vi "while循环的移位寄存器使用.vi"() -> ()   [LabVIEW 2019]
panel:
  out "数组 2":i32[](array[numeric])
  out "数组":i32[](array[numeric])
  out "数值 3":i32
  out "数值 2":i32
  out "数值":i32
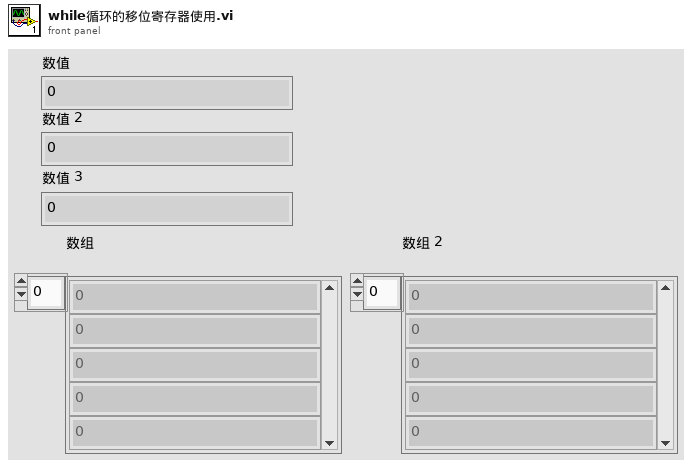
[diagram p1: front panel]
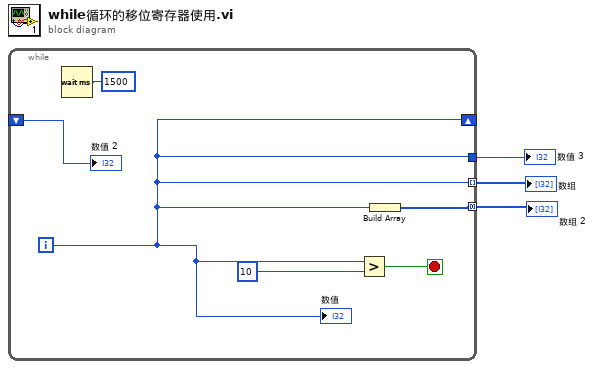
[diagram p0: block diagram]
diagram:
  n1 = while {
    shift-right: [w5] -> _
    shift-left: _ -> [w9]
    tunnel: [w5] -> w3
    tunnel: [w5] -> w2 mode=indexing
    tunnel: [w4] -> w1 mode=concatenating
    i -> [w5]
    stop <- w6 stop-if-true
    n2 = Wait (ms)(milliseconds to wait=u32 1500 ("等待时间（毫秒）")) -> ()  [unwired: 1 out]
    n3 = Greater?(x=w5, y=10) -> (0:w6:bool)
    n4 = Build Array(w5) -> (w4:i32[])
    "数值" <- w5
    "数值 2" <- w9
  }
  "数值 3" <- w3
  "数组" <- w2
  "数组 2" <- w1
